vi "Create RichText by Ref.vi"(8 "error in (no error)":errorcluster caption="错误输入（无错误）", 11 "RichTextBox":refnum<k24>(container)) -> (0 "error out":errorcluster caption="错误输出", 3 "RichText 输出":refnum<class "RichText.lvclass"> caption="DNL_LabVIEW Object out")   [LabVIEW 2012, in "RichText.lvclass"]
uses:
  RichText.lvclass
  RichText.lvclass/RichText.ctl
  System.Windows.Forms
panel:
  in  "RichText 输入":refnum<class "RichText.lvclass"> caption="DNL_LabVIEW Object in"
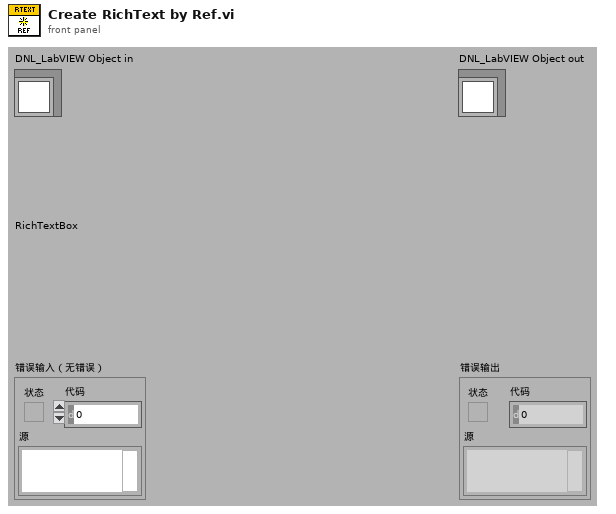
[diagram p1: front panel]
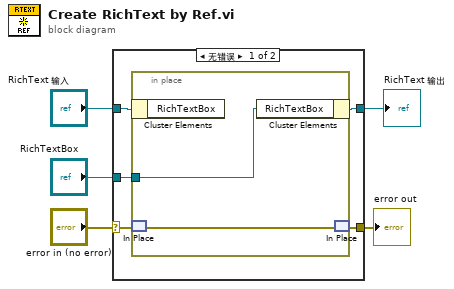
[diagram p0: block diagram]
diagram:
  n1 = case shown="无错误" "error in (no error)" {
    selector: "error in (no error)" -> [w7 w13]
    tunnel: [w8 w14] -> w3
    tunnel: "RichText 输入" -> [w10 w14]
    tunnel: "RichTextBox" -> [w9 _]
    tunnel: [w6 w13] -> w1
    frame No Error {
      n2 = in-place {
        in-place-border: w9 -> [w12]
        n3 = in-place-cluster #1(w10) -> ()  [unwired: 1 out]
        n4 = in-place-match #2(w7) -> (w11:errorcluster)
        n5 = in-place-cluster #1("RichTextBox"=w12) -> (w8:refnum<class "RichText.lvclass">)
        n6 = in-place-match #2(w11) -> (w6:errorcluster)
      }
    }
    frame Error {
    }
  }
  "error out" <- w1
  "RichText 输出" <- w3
